vi "Clear RTDriver VIs.vi"(8 "error in (no error)":errorcluster, 11 "Device Item Ref in in":T1 format="%.0x") -> (0 "error out":errorcluster, 3 "Device Item Ref out":T1 format="%.0x")   [LabVIEW 2019, in "TemplatePPL System Explorer.lvlib"]
uses:
  TemplatePPL System Explorer.lvlib
  <vilib>/NI VeriStand/Custom Device API/Custom Device Item Ref.ctl
  <vilib>/NI VeriStand/Custom Device API/Custom Device API.lvlib
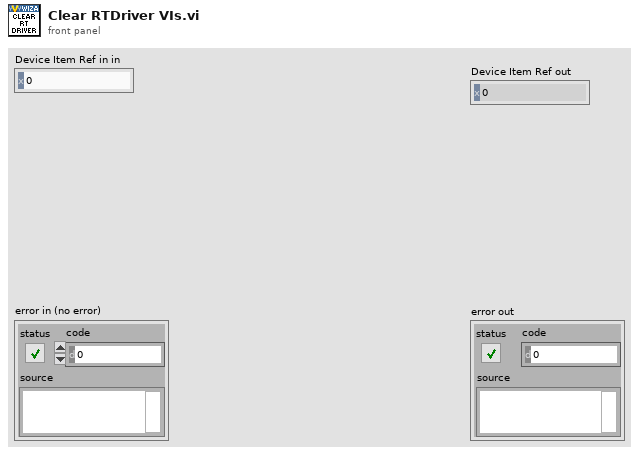
[diagram p1: front panel]
types:
  T1 = typedef "Custom Device API.lvlib/Custom Device Item Ref.ctl" = u64
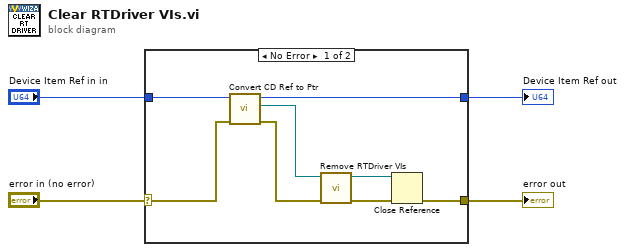
[diagram p0: block diagram]
diagram:
  n1 = case shown="No Error" "error in (no error)" {
    selector: "error in (no error)" -> [w10 w14]
    tunnel: "Device Item Ref in in" -> [w12 w13]
    tunnel: [w8 w13] -> w2
    tunnel: [w5 w14] -> w1
    frame No Error {
      n2 = call "Convert CD Ref to Ptr.vi"("error in (no error)"=w10, "Item Ref in"=w12) -> ("error out"=w9:errorcluster, ".NET Refnum out"=w11:refnum<k24>, "Item Ref out"=w8:T1)  [unwired: 7 in]
      n3 = call "Remove RTDriver VIs.vi"("error in (no error)"=w9, ".NET Refnum in"=w11) -> ("error out"=w7:errorcluster, ".NET Refnum out"=w6:refnum<k24>)  [unwired: 8 in]
      n4 = Close Reference(reference=w6, error in (no error)=w7) -> (error out=w5:errorcluster)
    }
    frame Error {
    }
  }
  "Device Item Ref out" <- w2
  "error out" <- w1
